vi "RichToFlatcif_launcher_LaunchConfig.vi"(5 "OutputClusterType":T1, 11 "InputCluster":T3) -> (3 "OutputCluster":T1)   [LabVIEW 2021, in "CIF_Launcher_server.lvlib"]
uses:
  CIF_Launcher_server.lvlib
  cif_launcher_LaunchConfig.ctl
  cif_manager_PluginName.ctl
  cif_launcher_LaunchConfig_Flat.ctl
  cif_manager_PluginName_Flat.ctl
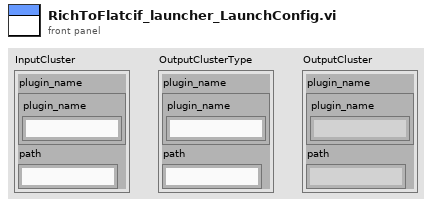
[diagram p1: front panel]
types:
  T1 = typedef "CIF_Launcher_server.lvlib/cif_launcher_LaunchConfig_Flat.ctl" = cluster{"plugin_name":T2, "path":string}
  T2 = typedef "CIF_Launcher_server.lvlib/cif_manager_PluginName_Flat.ctl" = cluster{"plugin_name":string}
  T3 = typedef "CIF_Launcher_server.lvlib/cif_launcher_LaunchConfig.ctl" = cluster{"plugin_name":T4, "path":string}
  T4 = typedef "CIF_Launcher_server.lvlib/cif_manager_PluginName.ctl" = cluster{"plugin_name":string}
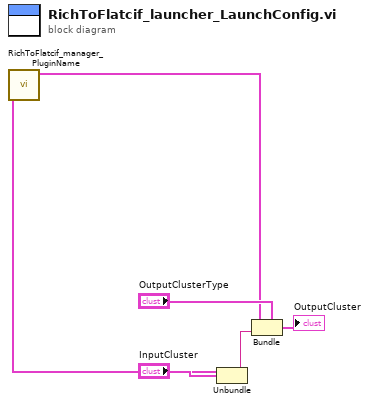
[diagram p0: block diagram]
diagram:
  n1 = Unbundle "Unbundle"("InputCluster") -> ("plugin_name"=w3:T4, "path"=w1:string)
  n2 = call "RichToFlatcif_manager_PluginName.vi"("InputCluster"=w3) -> ("OutputCluster"=w2:T2)  [unwired: 10 in]
  n3 = Bundle "Bundle"(cluster="OutputClusterType", "plugin_name"=w2, "path"=w1) -> (→"OutputCluster":T1)
